vi "from string.vi"(8 "error in":errorcluster, 9 "data":string, 10 "version":string, 11 "user tag bus module configuration In":refnum<class "TEST CONFIGURATION.lvclass">) -> (0 "error out":errorcluster, 3 "user tag bus module configuration Out":refnum<class "TEST CONFIGURATION.lvclass">)   [LabVIEW 2013, in "configuration tests.lvlib" / "TEST CONFIGURATION.lvclass"]
doc: "Provides an interface for loading a module configuration from a file or other serialized data source. It is recommended that all children of this class store data in two sets--data required for its own initialization, and any data required for parent initialization--and that each implementation uses the <b>Call Parent Method</b> primitive to de-serialize parent information. As a result, it is expected that every module configuration class calls <b>component configuration.lvclass:From String.vi</b>."
uses:
  TEST CONFIGURATION.lvclass
  state module configuration.ctl
  <vilib>/NI/Tag Bus Module Framework/channel/TBM channel.lvclass
  control module configuration.ctl
  gains.ctl
  <vilib>/NI/Tag Bus Module Framework/module configuration/TBM module configuration.lvclass
  TEST CONFIGURATION.lvclass/TEST CONFIGURATION.ctl
  <vilib>/NI/Configuration Framework/serializable configuration/NISE_CEF_serializable configuration.lvclass
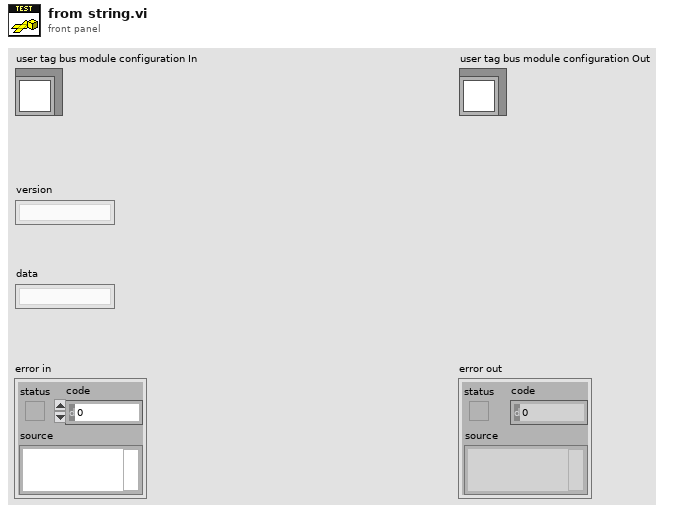
[diagram p1: front panel]
types:
  T1 = typedef "configuration tests.lvlib/TEST CONFIGURATION.lvclass/control module configuration.ctl" = cluster{"name":string, "setpoint":refnum<class "TBM channel.lvclass">, "process variable":refnum<class "TBM channel.lvclass">, "output":refnum<class "TBM channel.lvclass">, "gains":T2, "output range":cluster{"output high":dbl, "output low":dbl}}
  T2 = typedef "configuration tests.lvlib/TEST CONFIGURATION.lvclass/gains.ctl" = cluster{"Kp":dbl, "Ki":dbl, "Kd":dbl}
  T3 = typedef "configuration tests.lvlib/TEST CONFIGURATION.lvclass/state module configuration.ctl" = cluster{"fixed input":refnum<class "TBM channel.lvclass">, "fixed output":refnum<class "TBM channel.lvclass">, "initial state":u8}
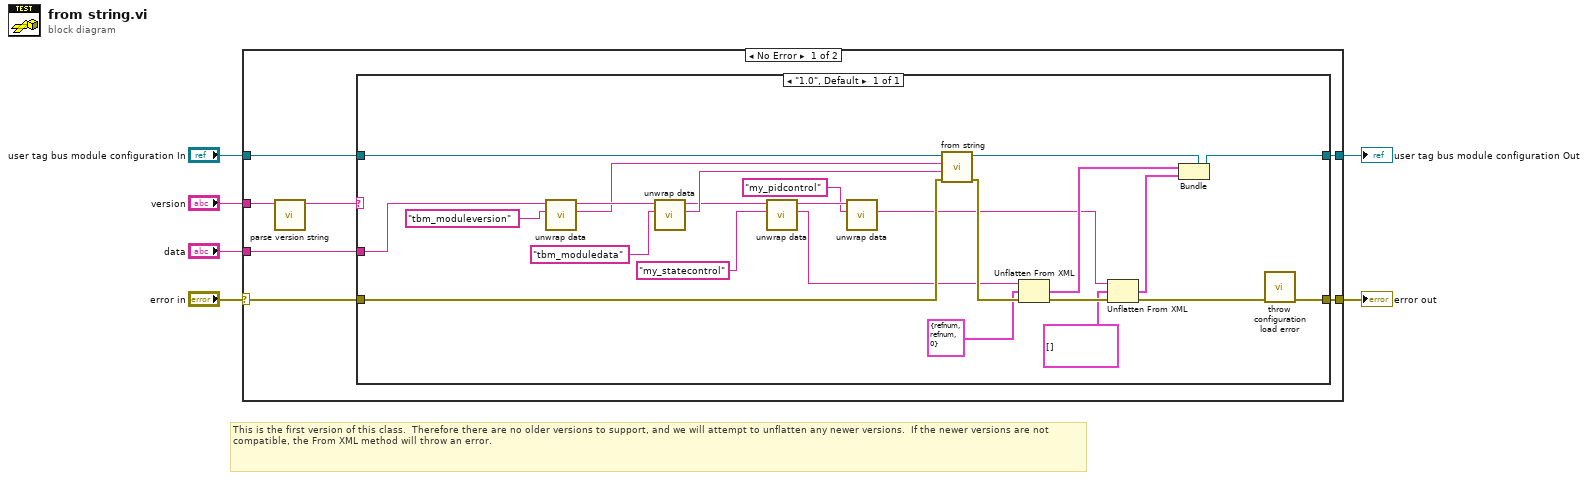
[diagram p0: block diagram]
diagram:
  # "This is the first version of this class.  Therefore there are no older versions to support, and we will attempt to unflatten any newer versions.  If the newer versions are not compatible, the From XML method will throw an error."
  n1 = case shown="No Error" "error in" {
    selector: "error in" -> [w7 w39]
    tunnel: "data" -> [w13 _]
    tunnel: "user tag bus module configuration In" -> [w12 w38]
    tunnel: [w11 w38] -> w5
    tunnel: [w10 w39] -> w4
    tunnel: "version" -> [w9 _]
    frame No Error {
      n2 = call <vilib>:"parse version string.vi"("full version"=w9) -> ("major.minor version"=w8:string)  [unwired: 7 in, 3 out]
      n3 = case shown="\"1.0\", Default" w8 {
        tunnel: w13 -> [w32]
        tunnel: w7 -> [w31]
        tunnel: w12 -> [w37]
        tunnel: [w26] -> w11
        tunnel: [w34] -> w10
        frame "1.0", Default {
          n4 = call <vilib>:"unwrap data.vi"("identifier"="tbm_moduleversion" ("additional identifier"), "data to unwrap"=w32) -> ("unwrapped data"=w27:string, "remaining string"=w33:string)  [unwired: 8 in]
          n5 = call <vilib>:"unwrap data.vi"("identifier"="tbm_moduledata" ("additional identifier"), "data to unwrap"=w33) -> ("unwrapped data"=w29:string, "remaining string"=w24:string)  [unwired: 8 in]
          n6 = call <vilib>:"unwrap data.vi"("identifier"="my_statecontrol" ("additional identifier"), "data to unwrap"=w24) -> ("unwrapped data"=w22:string, "remaining string"=w16:string)  [unwired: 8 in]
          n7 = call <vilib>:"unwrap data.vi"("identifier"="my_pidcontrol" ("additional identifier"), "data to unwrap"=w16) -> ("unwrapped data"=w14:string)  [unwired: 8 in, 1 out]
          n8 = call-parent "from string.vi"("error in"=w31, "data"=w29, "version"=w27, "module configuration in"=w37) -> ("error out"=w35:errorcluster, "module configuration out"=w36:refnum<class "TEST CONFIGURATION.lvclass">)  [unwired: 6 in]
          n9 = Unflatten From XML(xml string=w22, type=T3 {"fixed input"=refnum, "fixed output"=refnum, "initial state"=0} ("state module configuration"), error in (no error)=w35) -> (value=w19:T3, error out=w25:errorcluster)
          n10 = Unflatten From XML(xml string=w14, type=T1[] [] ("control functions"), error in (no error)=w25) -> (value=w17:T1[], error out=w21:errorcluster)
          n11 = Bundle(cluster=w36, w19, w17) -> (w26:refnum<class "TEST CONFIGURATION.lvclass">)
          n12 = call <vilib>:"throw configuration load error.vi"("error in"=w21) -> ("error out"=w34:errorcluster)  [unwired: 10 in]
        }
      }
    }
    frame Error {
    }
  }
  "error out" <- w4
  "user tag bus module configuration Out" <- w5
